vi "autoupdate_fiber_parameters_pixelmapper.vi"(8 "error in":errorcluster, 9 "Autoupdate":T3, 10 "Fiber parameters":T1={"Frequency"=2039.0, "Amplitude X"=0.3, "Amplitude Y"=0.3, "Initial Amplitude X"=0.0, "Initial Amplitude Y"=0.0, "Phase"=0.0, "Ramp type"=enum."Linear"} {"Phase" min=-90.0 max=90.0 step=5.0; "Initial Amplitude Y" min=0.0 max=1.0 step=0.1; "Initial Amplitude X" min=0.0 max=1.0 step=0.1; "Amplitude Y" min=0.0 max=4.0 step=0.1; "Amplitude X" min=0.0 max=4.0 step=0.1; "Frequency" min=100.0 max=6000.0 step=1.0}, 11 "Fiber parameters pixelmapper in":T1={"Frequency"=100.0, "Amplitude X"=0.0, "Amplitude Y"=0.0, "Initial Amplitude X"=0.0, "Initial Amplitude Y"=0.0, "Phase"=0.0, "Ramp type"=enum."Linear"} {"Phase" min=-90.0 max=90.0 step=5.0; "Initial Amplitude Y" min=0.0 max=1.0 step=0.1; "Initial Amplitude X" min=0.0 max=1.0 step=0.1; "Amplitude Y" min=0.0 max=4.0 step=0.1; "Amplitude X" min=0.0 max=4.0 step=0.1; "Frequency" min=100.0 max=6000.0 step=1.0}) -> (0 "error out":errorcluster, 3 "Fiber parameters pixelmapper out":T1={"Frequency"=100.0, "Amplitude X"=0.0, "Amplitude Y"=0.0, "Initial Amplitude X"=0.0, "Initial Amplitude Y"=0.0, "Phase"=0.0, "Ramp type"=enum."Linear"} {"Phase" min=-90.0 max=90.0 step=5.0; "Initial Amplitude Y" min=0.0 max=1.0 step=0.1; "Initial Amplitude X" min=0.0 max=1.0 step=0.1; "Amplitude Y" min=0.0 max=4.0 step=0.1; "Amplitude X" min=0.0 max=4.0 step=0.1; "Frequency" min=100.0 max=6000.0 step=1.0})   [LabVIEW 2011, in "Fiberscope_library.lvlib"]
uses:
  Fiberscope_library.lvlib
  typedefs/fiber_parameters_pixelmapper_autoupdate_cluster.ctl
  typedefs/fiber_parameters_cluster.ctl
  fpga/typedefs/ramp_type_enum.ctl
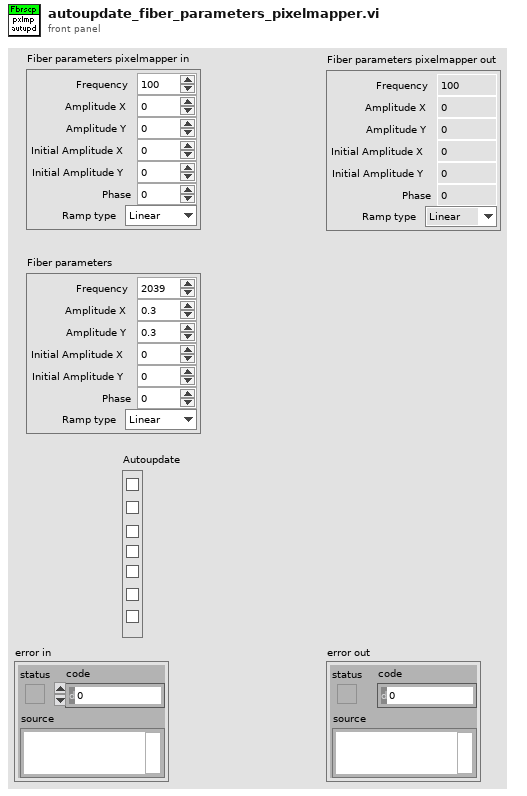
[diagram p1: front panel]
types:
  T1 = typedef "Fiberscope_library.lvlib/fiber_parameters_cluster.ctl" = cluster{"Frequency":dbl, "Amplitude X":dbl, "Amplitude Y":dbl, "Initial Amplitude X":dbl, "Initial Amplitude Y":dbl, "Phase":dbl, "Ramp type":T2}
  T2 = typedef "ramp_type_enum.ctl" = enum8{"Linear", "Sine"}
  T3 = typedef "Fiberscope_library.lvlib/fiber_parameters_pixelmapper_autoupdate_cluster.ctl" = cluster{"Frequency":bool, "Amplitude X":bool, "Amplitude Y":bool, "Initial Amplitude X":bool, "Initial Amplitude Y":bool, "Phase":bool, "Ramp type":bool}
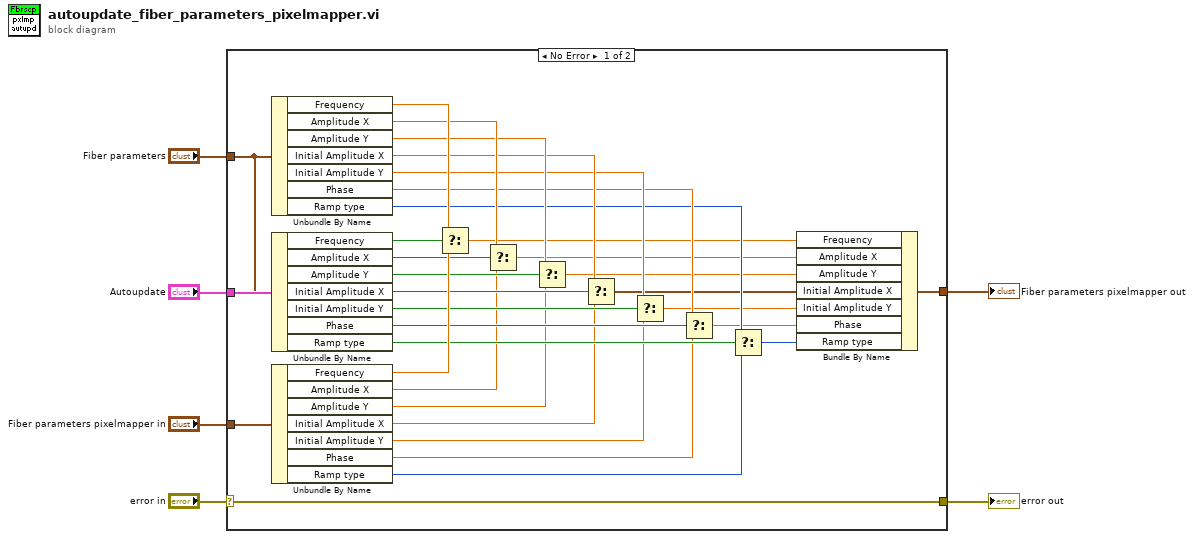
[diagram p0: block diagram]
diagram:
  n1 = case shown="No Error" "error in" {
    selector: "error in" -> [w39 w41]
    tunnel: [w39 w41] -> w5
    tunnel: "Fiber parameters pixelmapper in" -> [w38 _]
    tunnel: "Autoupdate" -> [w37 _]
    tunnel: "Fiber parameters" -> [w14 w40]
    tunnel: [w15 w40] -> w1
    frame No Error {
      n2 = Unbundle By Name(w14) -> ("Frequency"=w35:dbl, "Amplitude X"=w27:dbl, "Amplitude Y"=w25:dbl, "Initial Amplitude X"=w23:dbl, "Initial Amplitude Y"=w21:dbl, "Phase"=w19:dbl, "Ramp type"=w17:T2)
      n3 = Unbundle By Name(w37) -> ("Frequency"=w36:bool, "Amplitude X"=w33:bool, "Amplitude Y"=w32:bool, "Initial Amplitude X"=w31:bool, "Initial Amplitude Y"=w30:bool, "Phase"=w29:bool, "Ramp type"=w28:bool)
      n4 = Unbundle By Name(w38) -> ("Frequency"=w34:dbl, "Amplitude X"=w26:dbl, "Amplitude Y"=w24:dbl, "Initial Amplitude X"=w22:dbl, "Initial Amplitude Y"=w20:dbl, "Phase"=w18:dbl, "Ramp type"=w16:T2)
      n5 = Select(t=w35, s=w36, f=w34) -> (s? t:f=w13:dbl)
      n6 = Select(t=w27, s=w33, f=w26) -> (s? t:f=w12:dbl)
      n7 = Select(t=w25, s=w32, f=w24) -> (s? t:f=w11:dbl)
      n8 = Select(t=w23, s=w31, f=w22) -> (s? t:f=w10:dbl)
      n9 = Select(t=w21, s=w30, f=w20) -> (s? t:f=w9:dbl)
      n10 = Select(t=w19, s=w29, f=w18) -> (s? t:f=w8:dbl)
      n11 = Select(t=w17, s=w28, f=w16) -> (s? t:f=w7:T2)
      n12 = Bundle By Name(cluster=w14, "Frequency"=w13, "Amplitude X"=w12, "Amplitude Y"=w11, "Initial Amplitude X"=w10, "Initial Amplitude Y"=w9, "Phase"=w8, "Ramp type"=w7) -> (w15:T1)
    }
    frame Error {
    }
  }
  "error out" <- w5
  "Fiber parameters pixelmapper out" <- w1
